vi "Generate Assets Path.vi"() -> (0 "Assets path":path)   [LabVIEW 2018, in "Scripting API Unit Tests.lvclass"]
uses:
  Scripting API Unit Tests.lvclass
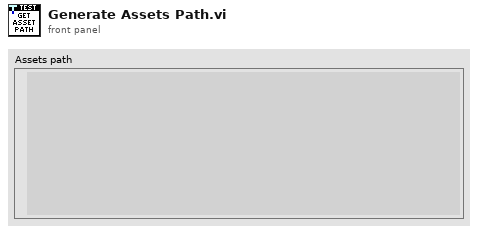
[diagram p1: front panel]
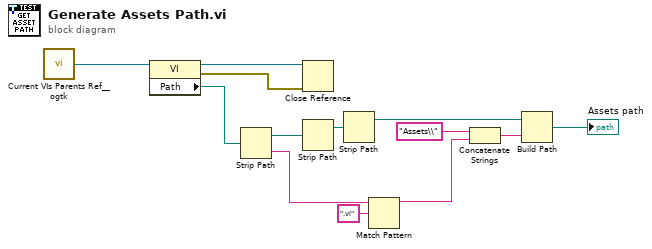
[diagram p0: block diagram]
diagram:
  n1 = call <userlib>:"Current VIs Parents Ref__ogtk.vi"() -> ("Calling VI's Reference"=w11:refnum<vi>)  [unwired: 2 in]
  n2 = property class="VI"(reference=w11) -> (reference out=w10:refnum<vi>, error out=w9:errorcluster, "Path"=w8:path)  [unwired: 1 in]
  n3 = Strip Path(path=w8) -> (stripped path=w13:path, name=w7:string)
  n4 = Close Reference(reference=w10, error in (no error)=w9) -> ()  [unwired: 1 out]
  n5 = Strip Path(path=w13) -> (stripped path=w12:path)  [unwired: 1 out]
  n6 = Strip Path(path=w12) -> (stripped path=w1:path)  [unwired: 1 out]
  n7 = Match Pattern(string=w7, regular expression=".vi") -> (before substring=w4:string)  [unwired: 1 in, 3 out]
  n8 = Concatenate Strings("Assets\\" ("string"), w4) -> (w2:string)
  n9 = Build Path(base path=w1, name or relative path=w2) -> (appended path=→"Assets path":path)
